vi "Read Number of Tatics.vi"(8 "error in (no error)":errorcluster, 11 "5RobotsRole in":refnum<class "5RobotsRole.lvclass">) -> (0 "error out":errorcluster, 2 "Number of Tatics":dbl=1.0, 3 "5RobotsRole out":refnum<class "5RobotsRole.lvclass">)   [LabVIEW 2020, in "5RobotsRole.lvclass"]
uses:
  5RobotsRole.lvclass
  5RobotsRole.lvclass/5RobotsRole.ctl
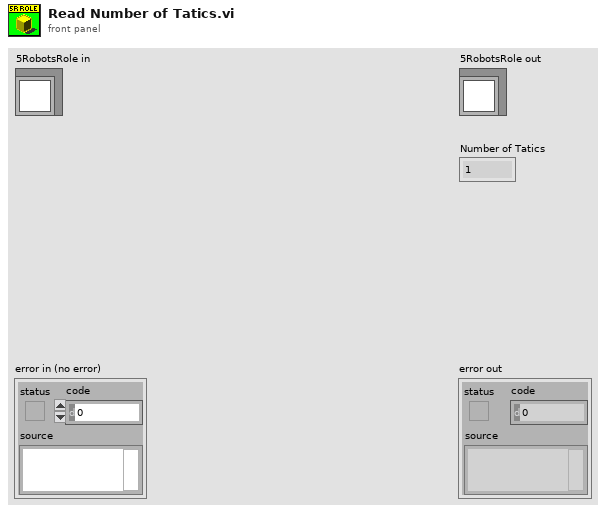
[diagram p1: front panel]
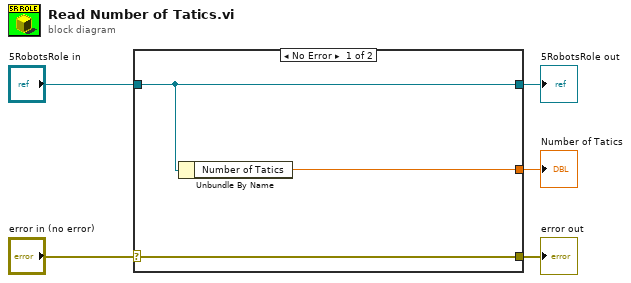
[diagram p0: block diagram]
diagram:
  n1 = case shown="No Error" "error in (no error)" {
    selector: "error in (no error)" -> [w8 w9]
    tunnel: [w8 w9] -> w4
    tunnel: [w7 w10] -> w2
    tunnel: "5RobotsRole in" -> [w7 w10]
    tunnel: [w6 _] -> w1
    frame No Error {
      n2 = Unbundle By Name(w7) -> ("Number of Tatics"=w6:dbl)
    }
    frame Error {
    }
  }
  "error out" <- w4
  "5RobotsRole out" <- w2
  "Number of Tatics" <- w1
